vi "FTW-TestExecutive-Core_Sequence_Start.vi"(0 "FTW-Scripter-Core In":refnum<class "FTW-TestExecutive-Core.lvclass">, 5 "Sequence":string, 11 "error in":errorcluster) -> (4 "FTW-Scripter-Core Out":refnum<class "FTW-TestExecutive-Core.lvclass">, 8 "Loaded Sequence":T1[](array[typedef]) {"Elapsed Time" format="%<%H:%M:%S%3u>t"}, 15 "error out":errorcluster)   [LabVIEW 2015]
uses:
  source/container/FTW-Container.lvclass
  FTW-TestExecutive_Step.ctl
  FTW-TestExecutive-Core.lvclass
  FTW-TestExecutive-Core_State.ctl
  FTW-TestExecutive-Core_Step_State.ctl
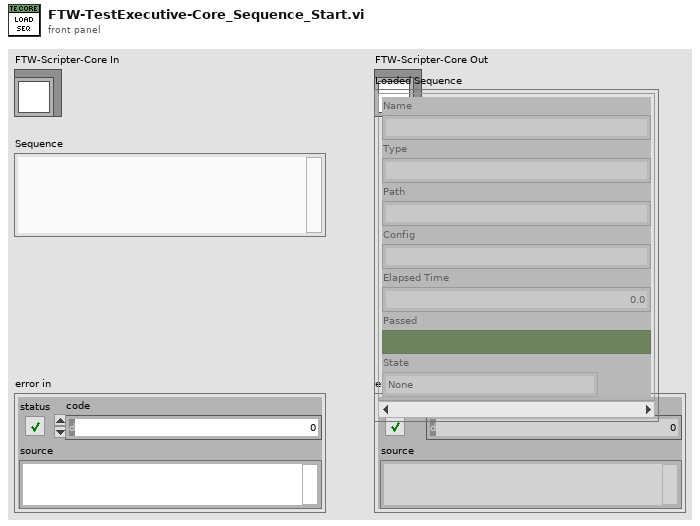
[diagram p1: front panel]
types:
  T1 = typedef "FTW-TestExecutive_Step.ctl" = cluster{"Name":string, "Type":string, "Path":string, "Config":string, "Elapsed Time":dbl, "Passed":bool, "State":T2}
  T2 = typedef "FTW-TestExecutive-Core_Step_State.ctl" = enum8{"None", "Failed", "Passed", "Timed out", "Aborted"}
  T3 = typedef "FTW-TestExecutive-Core.lvclass/FTW-TestExecutive-Core_State.ctl" = enum8{"Unloaded", "Loaded", "Executing", "Paused"}
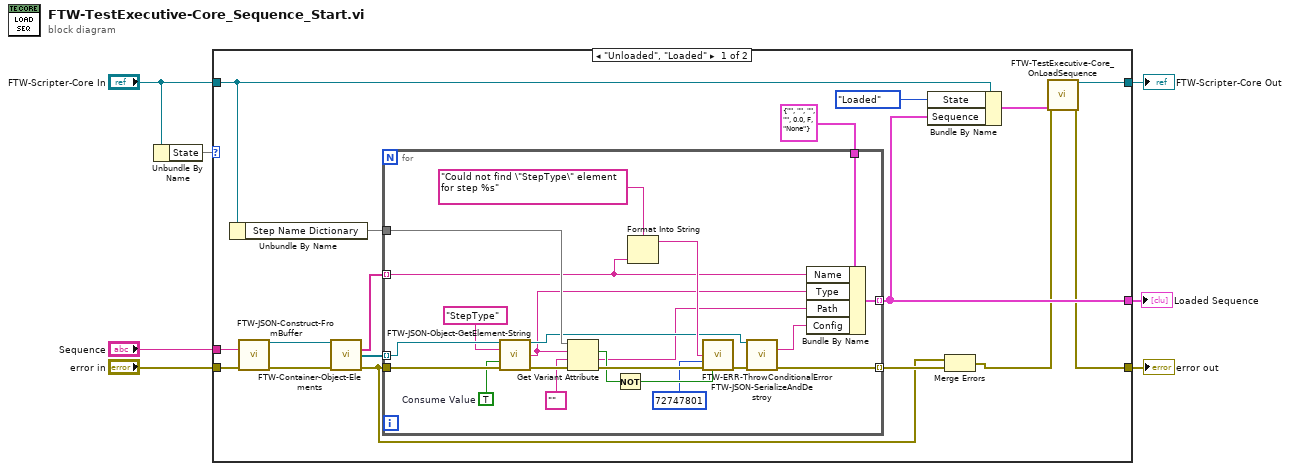
[diagram p0: block diagram]
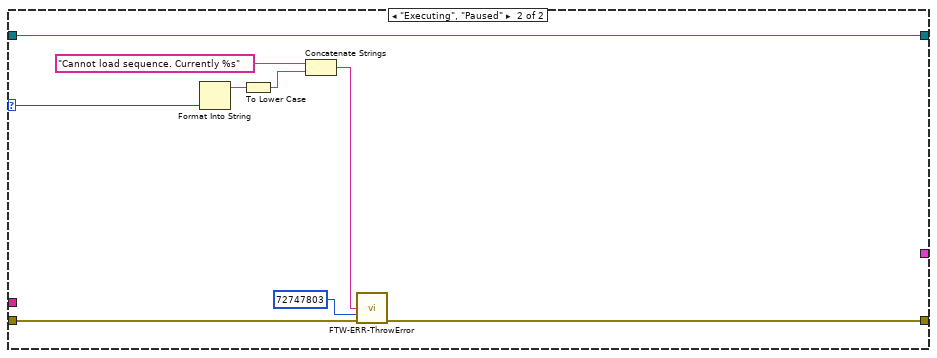
[diagram p2: hidden frame]
diagram:
  n1 = Unbundle By Name("FTW-Scripter-Core In") -> ("State"=w5)
  n2 = case shown="\"Unloaded\", \"Loaded\"" w5 {
    selector: w5 -> [_ w51]
    tunnel: [w10 w55] -> w7
    tunnel: "FTW-Scripter-Core In" -> [w13 w55]
    tunnel: [w8 w53] -> w4
    tunnel: "error in" -> [w24 w54]
    tunnel: "Sequence" -> [w20 _]
    tunnel: [w11 _] -> w1
    frame "Unloaded", "Loaded" {
      n3 = Unbundle By Name(w13) -> ("Step Name Dictionary"=w17)
      n4 = call "FTW-JSON-Construct-FromBuffer.vi"("JSON String (UTF-8)"=w20, "error in"=w24) -> ("JSON"=w19:refnum<class "FTW-Container.lvclass">, "error out"=w21:errorcluster)  [unwired: 12 in]
      n5 = call "FTW-Container-Object-Elements.vi"("FTW-Container In"=w19, "error in"=w21) -> ("Names"=w22:string[], "Object Elements"=w18:refnum<class "FTW-Container.lvclass">[], "error out"=w14:errorcluster)  [unwired: 10 in, 1 out]
      n6 = for {
        tunnel: w22 -> [w30] mode=indexing
        tunnel: w14 -> [w45]
        tunnel: w18 -> [w46] mode=indexing
        tunnel: w17 -> [w40]
        tunnel: [w32] -> w15 mode=indexing
        tunnel: [w29] -> w11 mode=indexing
        tunnel: T1 {"Name"="", "Type"="", "Path"="", "Config"="", "Elapsed Time"=0.0, "Passed"=FALSE, "State"=enum."None"} ("element") -> [w25]
        w43 = TRUE  # Consume Value
        n7 = call "FTW-JSON-Object-GetElement-String.vi"("JSON"=w46, "Key"="StepType", "Consume Value"=w43, "error in"=w45) -> ("JSON out"=w31:refnum<class "FTW-Container.lvclass">, "Value"=w27:string, "error out"=w42:errorcluster)  [unwired: 7 in, 2 out]
        n8 = Get Variant Attribute(Variant=w40, name=w27, default value (empty Variant)="" ("empty string"), error in=w42) -> (found=w37:bool, value=w26:string, error out=w39:errorcluster)  [unwired: 1 out]
        n9 = Not(x=w37) -> (.not. x?=w36:bool)
        n10 = Format Into String(format string="Could not find \"StepType\" element for step %s" ("Error Message"), w30) -> (resulting string=w34:string)  [unwired: 2 in, 1 out]
        n11 = call "FTW-ERR-ThrowConditionalError.vi"("Error Message"=w34, "Error Code"=72747801, "error in"=w39, "Throw Error?"=w36) -> ("error out"=w38:errorcluster)  [unwired: 11 in]
        n12 = call "FTW-JSON-SerializeAndDestroy.vi"("JSON"=w31, "error in"=w38) -> ("JSON String (UTF-8)"=w28:string, "error out"=w32:errorcluster)  [unwired: 12 in]
        n13 = Bundle By Name(cluster=w25, "Name"=w30, "Type"=w27, "Path"=w26, "Config"=w28) -> (w29:T1)
      }
      n14 = Bundle By Name(cluster=w13, "State"=FTW-TestExecutive-Core_State."Loaded", "Sequence"=w11) -> (w23:cluster{})
      n15 = Merge Errors(w14, w15) -> (w9:errorcluster)
      n16 = call "FTW-TestExecutive-Core_OnLoadSequence.vi"("FTW-Scripter-Core In"=w23, "error in"=w9) -> ("FTW-Scripter-Core Out"=w10:refnum<class "FTW-TestExecutive-Core.lvclass">, "error out"=w8:errorcluster)  [unwired: 12 in]
    }
    frame "Executing", "Paused" {
      n17 = Format Into String(w51) -> (resulting string=w50:string)  [unwired: 3 in, 1 out]
      n18 = To Lower Case(string=w50) -> (all lower case string=w48:string)
      n19 = Concatenate Strings("Cannot load sequence. Currently %s" ("Error Message"), w48) -> (w49:string)
      n20 = call "FTW-ERR-ThrowError.vi"("Error Message"=w49, "Error Code"=72747803, "error in"=w54) -> ("error out"=w53:errorcluster)  [unwired: 12 in]
    }
  }
  "FTW-Scripter-Core Out" <- w7
  "error out" <- w4
  "Loaded Sequence" <- w1
